vi "As NI Device.vi"(1 "IO Device":T1) -> (0 "As NI Device":i32)   [LabVIEW 2021, in "Load Frame.lvlib"]
doc: "Convert the Application's typedef value for a device to the corresponding DAQmx value."
uses:
  Load Frame.lvlib
  Acquisition/IO Device.ctl
  Acquisition/Acquisition.lvlib
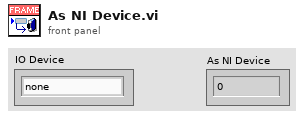
[diagram p1: front panel]
types:
  T1 = typedef "Acquisition.lvlib/IO Device.ctl" = enum16{"none", "9219", "9401"}
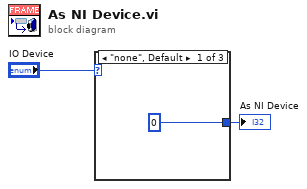
[diagram p0: block diagram]
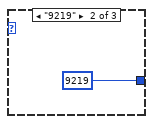
[diagram p2: hidden frame]
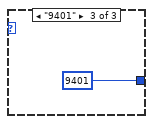
[diagram p3: hidden frame]
diagram:
  n1 = case shown="\"none\", Default" "IO Device" {
    tunnel: [0 9219 9401] -> w1
    frame "none", Default {
    }
    frame "9219" {
    }
    frame "9401" {
    }
  }
  "As NI Device" <- w1
